vi "write to board.vi"(7 "sync":refnum<k21>, 8 "clear":refnum<k21>, 9 "data":refnum<k21>, 10 "wright":refnum<k21>, 11 "Data":bool[](array[boolean])) -> (1 "Data Pin Task Out":refnum<k21>, 2 "Sync Pin Task Out":refnum<k21>, 3 "Refnum out":refnum<k21>, 4 "Clear Pin Task Out":refnum<k21>)   [LabVIEW 2020]
uses:
  <vilib>/DAQmx/write.llb/DAQmx Write (Digital Bool 1Line 1Point).vi
  <vilib>/DAQmx/miscellaneous.llb/DAQmx Fill In Error Info.vi
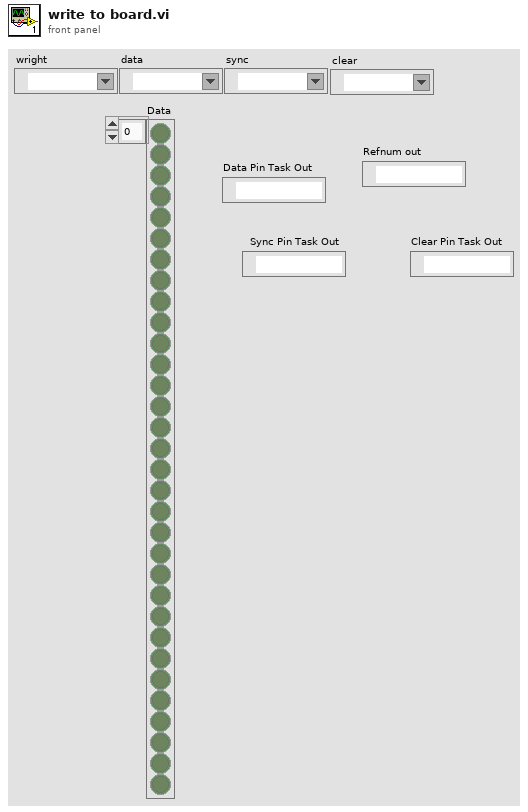
[diagram p1: front panel]
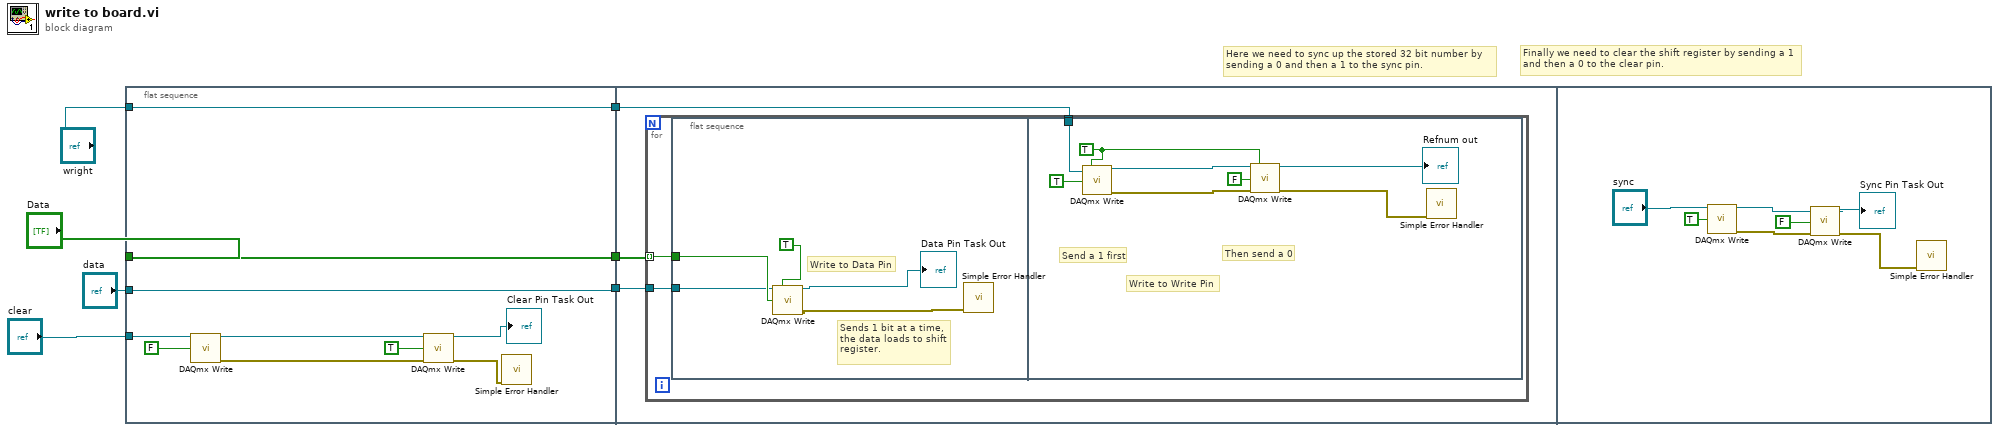
[diagram p0: block diagram]
diagram:
  # "Finally we need to clear the shift register by sending a 1\nand then a 0 to the clear pin."
  # "Here we need to sync up the stored 32 bit number by \nsending a 0 and then a 1 to the sync pin."
  n1 = flat-sequence {
    tunnel: "Data" -> [w17]
    tunnel: [w17] -> w7
    tunnel: "clear" -> [w10]
    tunnel: [w9] -> w4
    tunnel: "data" -> [w9]
    tunnel: [w8] -> w2
    tunnel: "wright" -> [w8]
    tunnel: w7 -> [w20]
    tunnel: w4 -> [w19]
    tunnel: w2 -> [w18]
    frame #0 {
      n2 = call-poly <vilib>:"DAQmx Write.vi"("task/channels in"=w10, "data"=FALSE) -> ("task out"=w14:refnum<k21>, "error out"=w13:errorcluster)  [unwired: 11 in, 1 out]
      n3 = call-poly <vilib>:"DAQmx Write.vi"("task/channels in"=w14, "data"=TRUE, "error in"=w13) -> ("task out"=→"Clear Pin Task Out":refnum<k21>, "error out"=w11:errorcluster)  [unwired: 10 in, 1 out]
      n4 = call <vilib>:"Simple Error Handler.vi"("error in (no error)"=w11) -> ()  [unwired: 4 in, 5 out]
    }
    frame #1 {
      n5 = for {
        tunnel: w20 -> [w23] mode=indexing
        tunnel: w19 -> [w22]
        tunnel: w18 -> [w21]
        n6 = flat-sequence {
          tunnel: w23 -> [w28]
          tunnel: w22 -> [w24]
          tunnel: w21 -> [w29]
          frame #0 {
            # "Sends 1 bit at a time,\nthe data loads to shift\nregister."
            # "Write to Data Pin"
            n7 = call-poly <vilib>:"DAQmx Write.vi"("task/channels in"=w24, "auto start"=TRUE, "data"=w28) -> ("task out"=→"Data Pin Task Out":refnum<k21>, "error out"=w25:errorcluster)  [unwired: 10 in, 1 out]
            n8 = call <vilib>:"Simple Error Handler.vi"("error in (no error)"=w25) -> ()  [unwired: 4 in, 5 out]
          }
          frame #1 {
            w30 = TRUE
            # "Then send a 0"
            # "Send a 1 first"
            # "Write to Write Pin"
            n9 = call-poly <vilib>:"DAQmx Write.vi"("task/channels in"=w29, "auto start"=w30, "data"=TRUE) -> ("task out"=w31:refnum<k21>, "error out"=w32:errorcluster)  [unwired: 10 in, 1 out]
            n10 = call-poly <vilib>:"DAQmx Write.vi"("task/channels in"=w31, "auto start"=w30, "data"=FALSE, "error in"=w32) -> ("task out"=→"Refnum out":refnum<k21>, "error out"=w33:errorcluster)  [unwired: 9 in, 1 out]
            n11 = call <vilib>:"Simple Error Handler.vi"("error in (no error)"=w33) -> ()  [unwired: 4 in, 5 out]
          }
        }
      }
    }
    frame #2 {
      n12 = call-poly <vilib>:"DAQmx Write.vi"("task/channels in"="sync", "data"=TRUE) -> ("task out"=w38:refnum<k21>, "error out"=w39:errorcluster)  [unwired: 11 in, 1 out]
      n13 = call-poly <vilib>:"DAQmx Write.vi"("task/channels in"=w38, "data"=FALSE, "error in"=w39) -> ("task out"=→"Sync Pin Task Out":refnum<k21>, "error out"=w40:errorcluster)  [unwired: 10 in, 1 out]
      n14 = call <vilib>:"Simple Error Handler.vi"("error in (no error)"=w40) -> ()  [unwired: 4 in, 5 out]
    }
  }
